vi "雷达回波模拟信号产生.vi"(11 "槽位号":i16) -> ()   [LabVIEW 2011]
doc: "打开板卡操作，输出板卡句柄！当有多个板卡时，根据板卡索引号打开不同板卡！\n如果同时使用一块板卡的多种功能，可将输出句柄连接到不同的功能任务中。\n此VI是创建所有任务的前提！"
uses:
  _SubVI/dll/P3060.dll
panel:
  in  "加载程序":bool caption="确定按钮"
  in  "取消按钮":bool
  out "error out":errorcluster caption="错误输出"
  in  "确定按钮":bool
  in  "开关十":bool=TRUE
  in  "开关九":bool=TRUE
  in  "开关八":bool=TRUE
  in  "开关七":bool=TRUE
  in  "开关六":bool=TRUE
  in  "开关五":bool=TRUE
  in  "开关四":bool=TRUE
  in  "开关三":bool=TRUE
  in  "开关二":bool=TRUE
  in  "开关一":bool=TRUE
  in  "延时十":dbl=2.0 min=0.02 max=20.0 step=0.02
  in  "延时九":dbl=2.0 min=0.02 max=20.0 step=0.02
  in  "延时八":dbl=2.0 min=0.02 max=20.0 step=0.02
  in  "延时七":dbl=2.0 min=0.02 max=20.0 step=0.02
  in  "延时六":dbl=2.0 min=0.02 max=20.0 step=0.02
  in  "延时五":dbl=2.0 min=0.02 max=20.0 step=0.02
  in  "延时四":dbl=2.0 min=0.02 max=20.0 step=0.02
  in  "延时三":dbl=2.0 min=0.02 max=20.0 step=0.02
  in  "延时二":dbl=2.0 min=0.02 max=20.0 step=0.02
  in  "延时一":dbl=2.0 min=0.02 max=20.0 step=0.02
  in  "多谱勒频率十":dbl=450000.0
  in  "多谱勒频率九":dbl=400000.0
  in  "多谱勒频率八":dbl=350000.0
  in  "多谱勒频率七":dbl=300000.0
  in  "多谱勒频率六":dbl=250000.0
  in  "多谱勒频率五":dbl=200000.0
  in  "多谱勒频率四":dbl=150000.0
  in  "多谱勒频率三":dbl=100000.0
  in  "多谱勒频率二":dbl=50000.0
  in  "多谱勒频率一":dbl
  # "us"
  # "Hz"
  # "us"
  # "Hz"
  # "us"
  # "Hz"
  # "us"
  # "Hz"
  # "us"
  # "Hz"
  # "us"
  # "Hz"
  # "us"
  # "Hz"
  # "us"
  # "Hz"
  # "us"
  # "Hz"
  # "us"
  # "Hz"
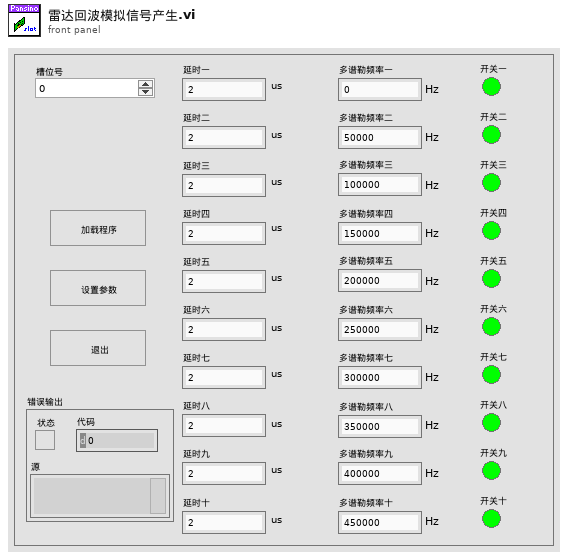
[diagram p1: front panel]
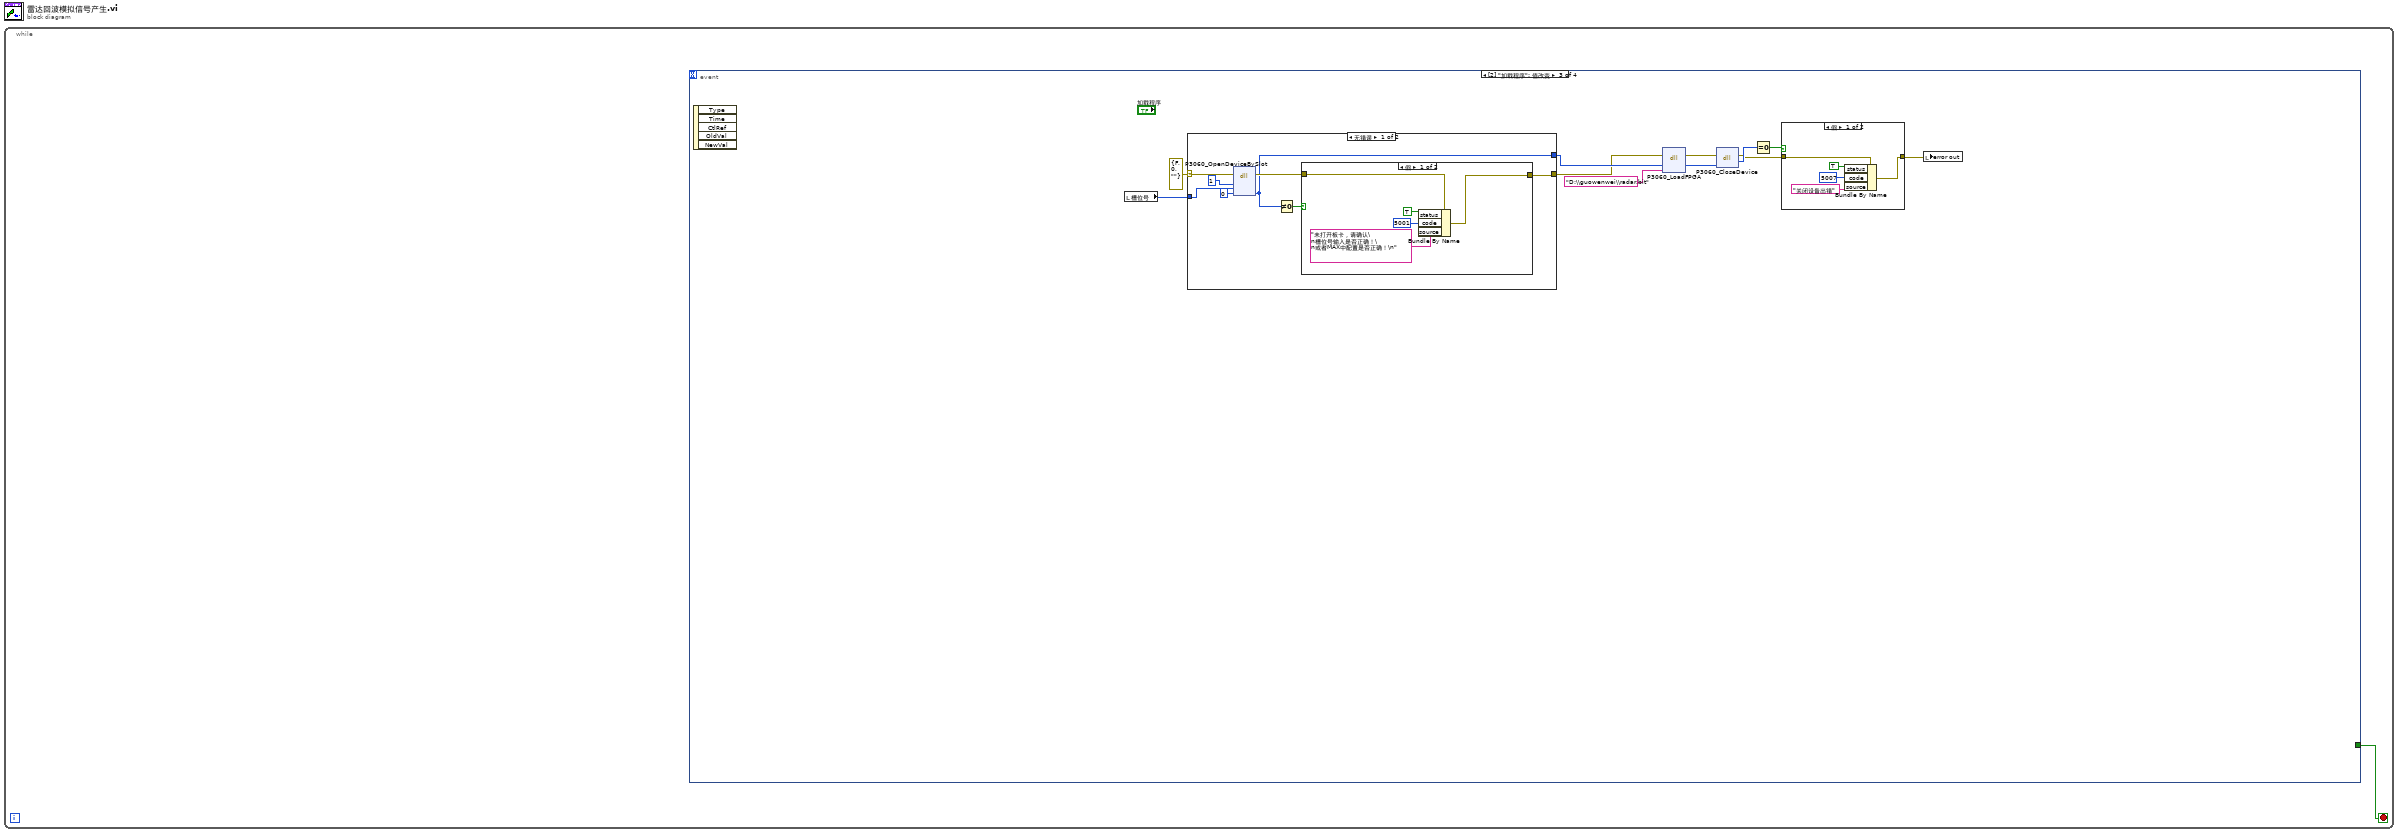
[diagram p0: block diagram]
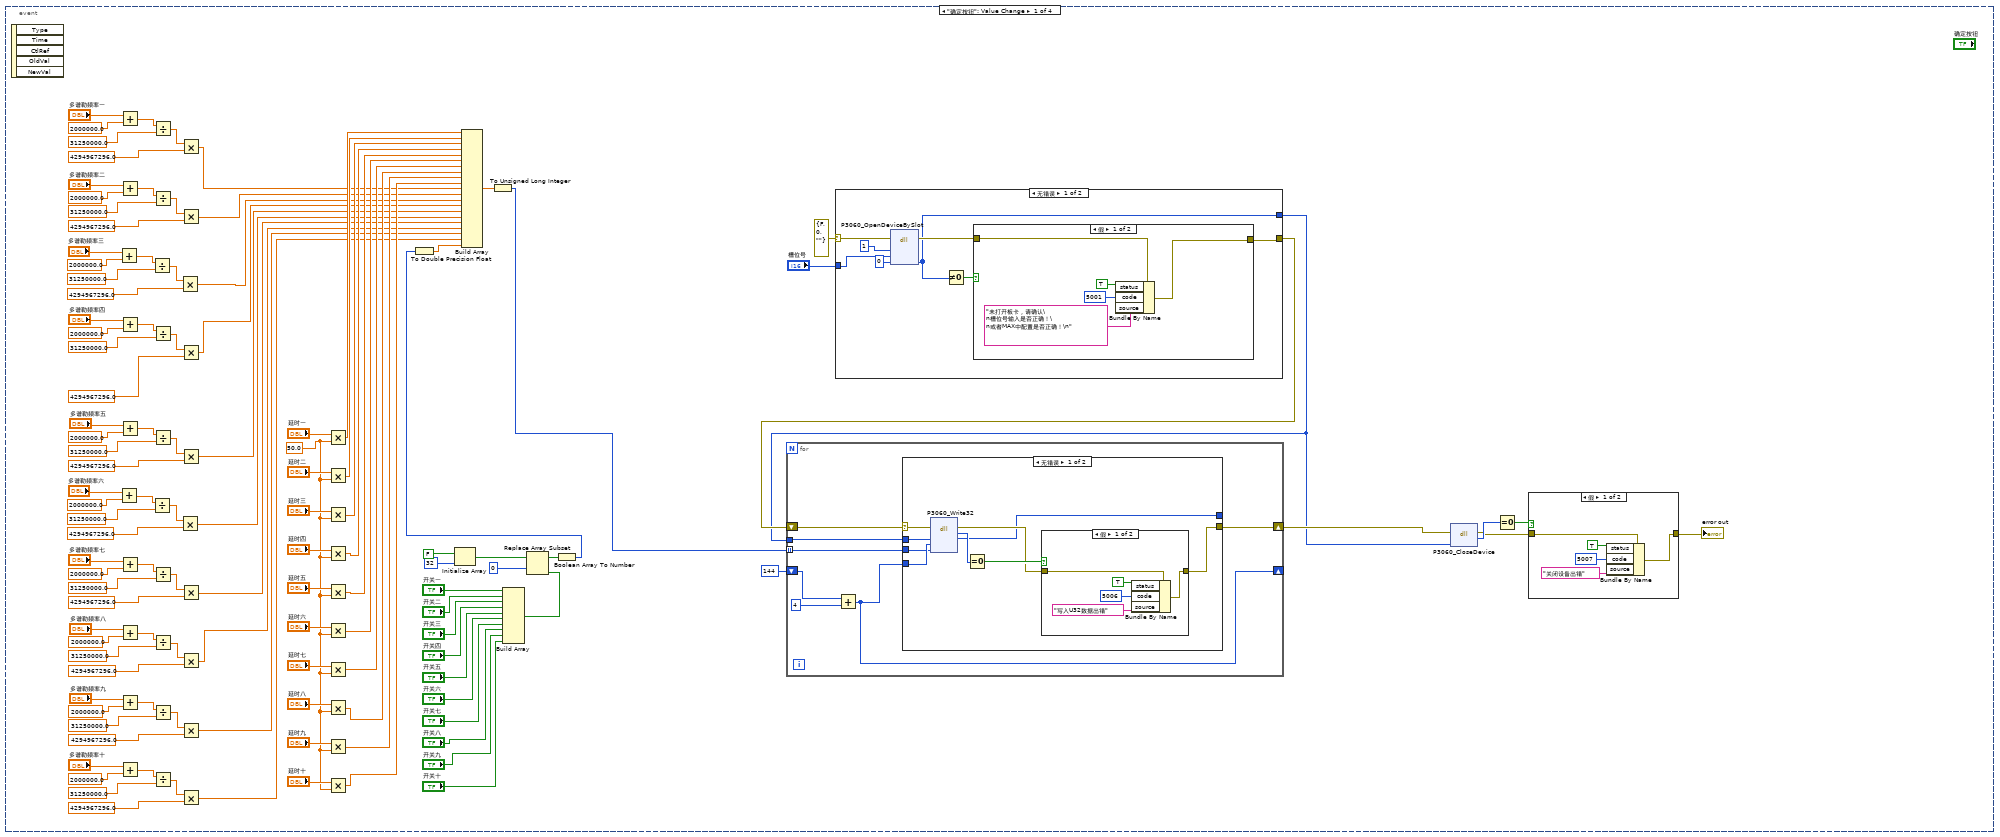
[diagram p2: hidden frame]
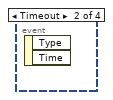
[diagram p8: hidden frame]
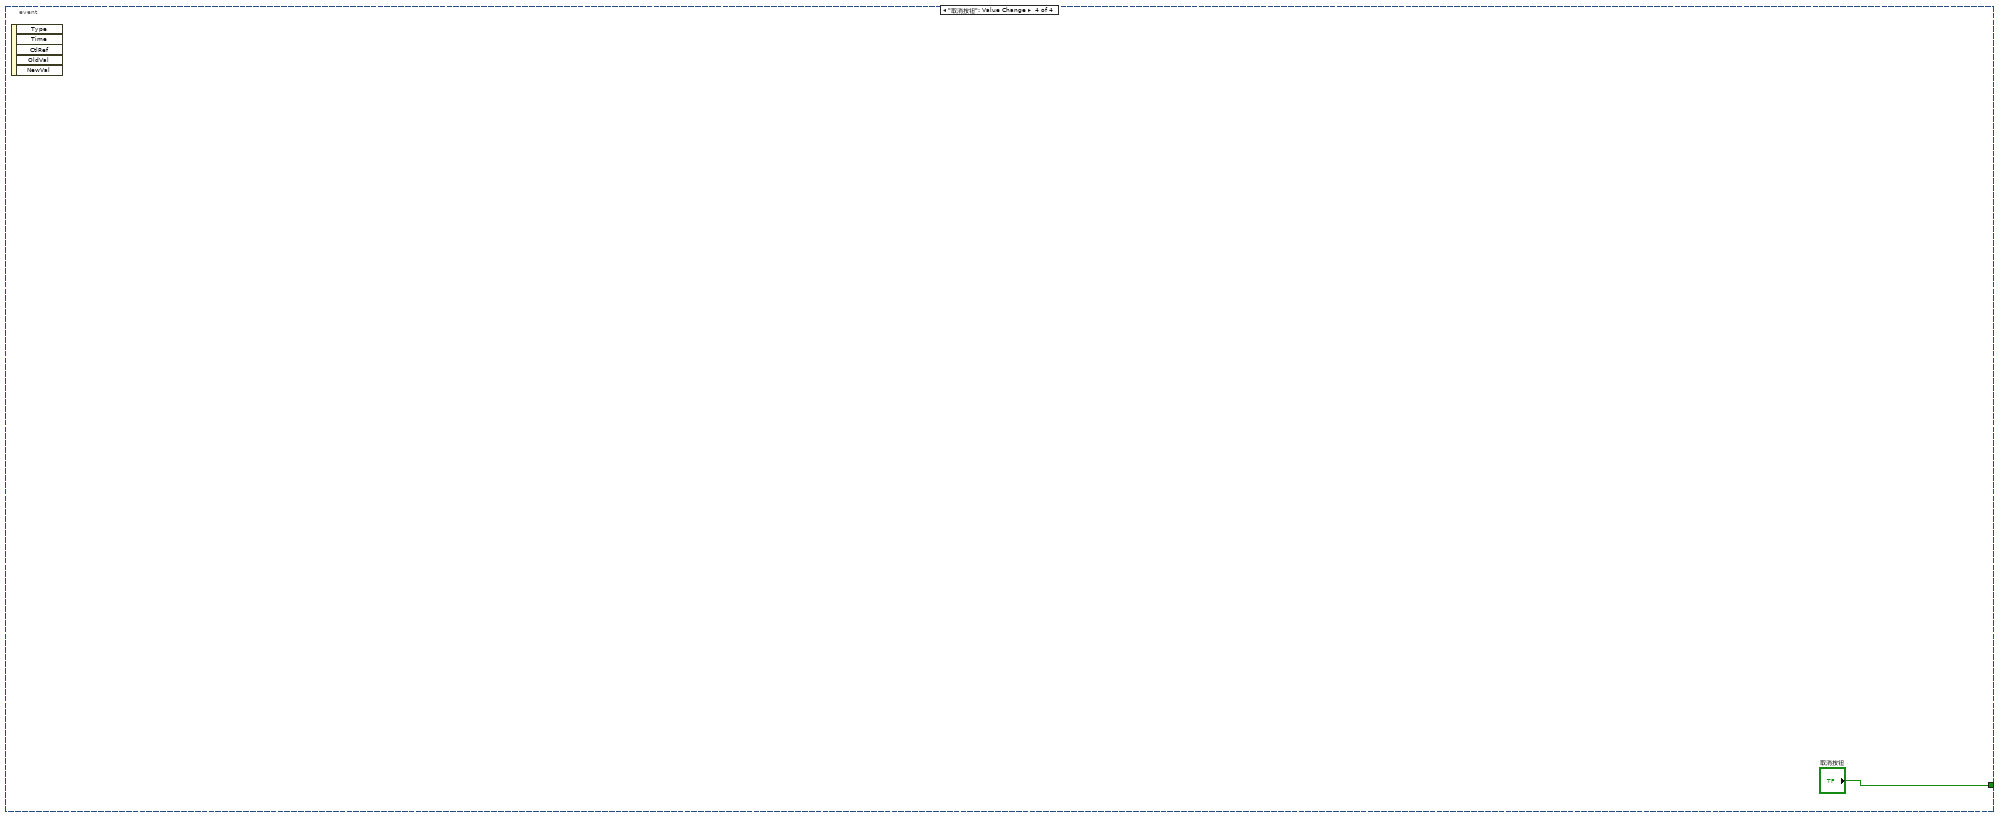
[diagram p12: hidden frame]
diagram:
  n1 = while {
    stop <- w1 stop-if-true
    n2 = event shown="[2] \"加载程序\": 值改变" {
      selector: _ -> [_ _ _ _]
      dyn-events: _ -> [_ _ _ _]
      timeout: _ -> [_ _ _ _]
      tunnel: [_ _ _ "取消按钮"] -> w1
      event "确定按钮": Value Change {
        w45 = 50.0 ("y")
        n3 = event-data() -> ()  [unwired: 1 in, 5 out]
        n4 = Add(x="多谱勒频率三", y=2000000.0) -> (x+y=w101:dbl)
        n5 = Add(x="多谱勒频率六", y=2000000.0) -> (x+y=w86:dbl)
        n6 = Add(x="多谱勒频率一", y=2000000.0) -> (x+y=w112:dbl)
        n7 = Add(x="多谱勒频率二", y=2000000.0) -> (x+y=w107:dbl)
        n8 = Add(x="多谱勒频率四", y=2000000.0) -> (x+y=w96:dbl)
        n9 = Add(x="多谱勒频率五", y=2000000.0) -> (x+y=w91:dbl)
        n10 = Add(x="多谱勒频率七", y=2000000.0) -> (x+y=w81:dbl)
        n11 = Add(x="多谱勒频率十", y=2000000.0) -> (x+y=w66:dbl)
        n12 = Add(x="多谱勒频率八", y=2000000.0) -> (x+y=w76:dbl)
        n13 = Add(x="多谱勒频率九", y=2000000.0) -> (x+y=w71:dbl)
        n14 = Divide(x=w101, y=31250000.0) -> (x/y=w99:dbl)
        n15 = Divide(x=w86, y=31250000.0) -> (x/y=w84:dbl)
        n16 = Divide(x=w112, y=31250000.0) -> (x/y=w110:dbl)
        n17 = Divide(x=w107, y=31250000.0) -> (x/y=w105:dbl)
        n18 = Divide(x=w96, y=31250000.0) -> (x/y=w94:dbl)
        n19 = Divide(x=w91, y=31250000.0) -> (x/y=w89:dbl)
        n20 = Divide(x=w81, y=31250000.0) -> (x/y=w79:dbl)
        n21 = Divide(x=w66, y=31250000.0) -> (x/y=w64:dbl)
        n22 = Divide(x=w76, y=31250000.0) -> (x/y=w74:dbl)
        n23 = Divide(x=w71, y=31250000.0) -> (x/y=w69:dbl)
        n24 = Multiply(x=w99, y=4294967296.0) -> (x*y=w14:dbl)
        n25 = Multiply(x=w84, y=4294967296.0) -> (x*y=w17:dbl)
        n26 = Multiply(x=w110, y=4294967296.0) -> (x*y=w12:dbl)
        n27 = Multiply(x=w105, y=4294967296.0) -> (x*y=w13:dbl)
        n28 = Multiply(x=w94, y=4294967296.0) -> (x*y=w15:dbl)
        n29 = Multiply(x=w89, y=4294967296.0) -> (x*y=w16:dbl)
        n30 = Multiply(x=w79, y=4294967296.0) -> (x*y=w18:dbl)
        n31 = Multiply(x=w64, y=4294967296.0) -> (x*y=w21:dbl)
        n32 = Multiply(x=w74, y=4294967296.0) -> (x*y=w19:dbl)
        n33 = Multiply(x=w69, y=4294967296.0) -> (x*y=w20:dbl)
        n34 = Multiply(x="延时一", y=w45) -> (x*y=w31:dbl)
        n35 = Multiply(x="延时二", y=w45) -> (x*y=w30:dbl)
        n36 = Multiply(x="延时三", y=w45) -> (x*y=w29:dbl)
        n37 = Multiply(x="延时四", y=w45) -> (x*y=w28:dbl)
        n38 = Multiply(x="延时五", y=w45) -> (x*y=w27:dbl)
        n39 = Multiply(x="延时六", y=w45) -> (x*y=w26:dbl)
        n40 = Multiply(x="延时七", y=w45) -> (x*y=w25:dbl)
        n41 = Multiply(x="延时八", y=w45) -> (x*y=w24:dbl)
        n42 = Multiply(x="延时九", y=w45) -> (x*y=w23:dbl)
        n43 = Multiply(x="延时十", y=w45) -> (x*y=w22:dbl)
        n44 = Initialize Array(FALSE, 32 ("维数大小")) -> (w118:bool[])
        n45 = Build Array("开关一", "开关二", "开关三", "开关四", "开关五", "开关六", "开关七", "开关八", "开关九", "开关十") -> (w119:bool[])
        n46 = Replace Array Subset(array=w118, new element=w119, index=0 ("索引")) -> (w116:bool[])
        n47 = Boolean Array To Number(Boolean array=w116) -> (number=w32:u32)
        n48 = To Double Precision Float(number=w32) -> (double precision float=w33:dbl)
        n49 = Build Array(w31, w30, w29, w28, w27, w26, w25, w24, w23, w22, w12, w13, w14, w15, w16, w17, w18, w19, w20, w21, w33) -> (w34:dbl[])
        n50 = To Unsigned Long Integer(number=w34) -> (unsigned 32bit integer=w35:u32[])
        n51 = case shown="无错误" errorcluster {"status"=FALSE, "code"=0, "source"=""} ("error IO") {
          selector: errorcluster {"status"=FALSE, "code"=0, "source"=""} ("error IO") -> [w160 w167]
          tunnel: [w156 w167] -> w10
          tunnel: "槽位号" -> [w159 _]
          tunnel: [w155 _] -> w3
          frame No Error {
            n52 = dll-call lib="PTH1_abs D\tguowenwei\tDAC测试P3060P3060\nP3060APILVLabviewP3060_SubVIdll\tP3060.dll" fn="P3060_OpenDeviceBySlot"(error in=w160, "Classis"=i16 1, "槽位号"=w159, "设备句柄"=0) -> (error out=w157:errorcluster, "设备句柄"=w155:i32)  [unwired: 5 in, 1 out]
            n53 = Not Equal To 0?(x=w155) -> (x != 0?=w158:bool)
            n54 = case shown="假" w158 {
              tunnel: w157 -> [w165 w166]
              tunnel: [w161 w166] -> w156
              frame False {
                n55 = Bundle By Name(cluster=w165, "status"=TRUE, "code"=5001, "source"="未打开板卡，请确认\n槽位号输入是否正确！\n或者MAX中配置是否正确！\n") -> (w161:errorcluster)
              }
              frame True {
              }
            }
          }
          frame Error {
          }
        }
        n56 = for {
          tunnel: w3 -> [w134]
          tunnel: w35 -> [w133] mode=indexing
          shift-right: [w131] -> _
          shift-left: u32 144 ("偏移地址") -> [w132]
          shift-right: [w129] -> w4
          shift-left: w10 -> [w135]
          n57 = Add(x=w132, y=4 ("x")) -> (x+y=w131:u32)
          n58 = case shown="无错误" w135 {
            selector: w135 -> [w140 w152]
            tunnel: [w144 w152] -> w129
            tunnel: w134 -> [w139 w151]
            tunnel: w131 -> [w138 _]
            tunnel: [w137 w151] -> _
            tunnel: w133 -> [w136 _]
            frame No Error {
              n59 = dll-call lib="PTH1_abs D\tguowenwei\tDAC测试P3060P3060\nP3060APILVLabviewP3060_SubVIdll\tP3060.dll" fn="P3060_Write32"(error in=w140, "hDev"=w139, "Offset"=w138, "data"=w136) -> (error out=w141:errorcluster, "return"=w143:i32, "hDev"=w137:i32)  [unwired: 4 in, 1 out]
              n60 = Equal To 0?(x=w143) -> (x = 0?=w142:bool)
              n61 = case shown="假" w142 {
                tunnel: [w148 w150] -> w144
                tunnel: w141 -> [w149 w150]
                frame False {
                  n62 = Bundle By Name(cluster=w149, "status"=TRUE, "code"=5006, "source"="写入U32数据出错") -> (w148:errorcluster)
                }
                frame True {
                }
              }
            }
            frame Error {
            }
          }
        }
        n63 = dll-call lib="PTH1_abs D\tguowenwei\tDAC测试P3060P3060\nP3060APILVLabviewP3060_SubVIdll\tP3060.dll" fn="P3060_CloseDevice"(error in=w4, "hDev"=w3) -> (error out=w5:errorcluster, "hDevOut"=w7:i32)  [unwired: 3 in, 1 out]
        n64 = Equal To 0?(x=w7) -> (x = 0?=w6:bool)
        n65 = case shown="假" w6 {
          tunnel: [w126 w128] -> w8
          tunnel: w5 -> [w127 w128]
          frame False {
            n66 = Bundle By Name(cluster=w127, "status"=TRUE, "code"=5007, "source"="关闭设备出错") -> (w126:errorcluster)
          }
          frame True {
          }
        }
        "error out" <- w8
      }
      event Timeout {
        n67 = event-data() -> ()  [unwired: 1 in, 2 out]
      }
      event "加载程序": Value Change {
        n68 = event-data() -> ()  [unwired: 1 in, 5 out]
        n69 = local read "槽位号"() -> (w175:i16)
        n70 = case shown="无错误" errorcluster {"status"=FALSE, "code"=0, "source"=""} ("error IO") {
          selector: errorcluster {"status"=FALSE, "code"=0, "source"=""} ("error IO") -> [w192 w199]
          tunnel: [w188 w199] -> w171
          tunnel: w175 -> [w191 _]
          tunnel: [w187 _] -> w177
          frame No Error {
            n71 = dll-call lib="PTH1_abs D\tguowenwei\tDAC测试P3060P3060\nP3060APILVLabviewP3060_SubVIdll\tP3060.dll" fn="P3060_OpenDeviceBySlot"(error in=w192, "Classis"=i16 1, "槽位号"=w191, "设备句柄"=0) -> (error out=w189:errorcluster, "设备句柄"=w187:i32)  [unwired: 5 in, 1 out]
            n72 = Not Equal To 0?(x=w187) -> (x != 0?=w190:bool)
            n73 = case shown="假" w190 {
              tunnel: w189 -> [w197 w198]
              tunnel: [w193 w198] -> w188
              frame False {
                n74 = Bundle By Name(cluster=w197, "status"=TRUE, "code"=5001, "source"="未打开板卡，请确认\n槽位号输入是否正确！\n或者MAX中配置是否正确！\n") -> (w193:errorcluster)
              }
              frame True {
              }
            }
          }
          frame Error {
          }
        }
        n75 = dll-call lib="PTH1_abs D\tguowenwei\tDAC测试P3060P3060\nP3060APILVLabviewP3060_SubVIdll\tP3060.dll" fn="P3060_LoadFPGA"(error in=w171, "hDev"=w177, "filepath"="D:\\guowenwei\\radar.bit") -> (error out=w170:errorcluster, "hDev"=w169:i32)  [unwired: 4 in, 1 out]
        n76 = dll-call lib="PTH1_abs D\tguowenwei\tDAC测试P3060P3060\nP3060APILVLabviewP3060_SubVIdll\tP3060.dll" fn="P3060_CloseDevice"(error in=w170, "hDev"=w169) -> (error out=w172:errorcluster, "hDevOut"=w174:i32)  [unwired: 3 in, 1 out]
        n77 = Equal To 0?(x=w174) -> (x = 0?=w173:bool)
        n78 = case shown="假" w173 {
          tunnel: [w182 w184] -> w168
          tunnel: w172 -> [w183 w184]
          frame False {
            n79 = Bundle By Name(cluster=w183, "status"=TRUE, "code"=5007, "source"="关闭设备出错") -> (w182:errorcluster)
          }
          frame True {
          }
        }
        n80 = local write "error out"(w168) -> ()
      }
      event "取消按钮": Value Change {
        n81 = event-data() -> ()  [unwired: 1 in, 5 out]
      }
    }
  }
